vi "Read Simulation Sonar ID.vi"(5 "Ping DIO Channel":T1=enum."DIO 1", 9 "Echo DIO Channel":T1=enum."DIO 2") -> (8 "sonar ID":string, 10 "success?":bool)   [LabVIEW 2017]
uses:
  <vilib>/Rock Robotics/SystemInterfaces/DIO/FPGA_DIOChannel.ctl
panel:
  out "String":string
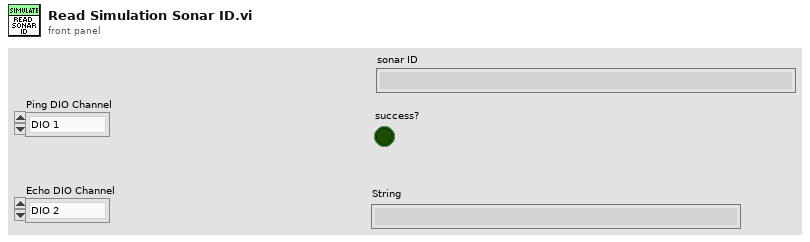
[diagram p1: front panel]
types:
  T1 = typedef "FPGA_DIOChannel.ctl" = enum8{"DIO 0", "DIO 1", "DIO 2", "DIO 3", "DIO 4", "DIO 5", "DIO 6", "DIO 7", "DIO 8", "DIO 9", "DIO MXP 0", "DIO MXP 1", "DIO MXP 2", "DIO MXP 3", "DIO MXP 4", "DIO MXP 5", "DIO MXP 6", "DIO MXP 7", "DIO MXP 8", "DIO MXP 9", "DIO MXP 10", "DIO MXP 11", "DIO MXP 12", "DIO MXP 13", "DIO MXP 14", "DIO MXP 15", "SPI Port CS1", "SPI Port CS2", "SPI Port CS3", "SPI Port MISO", "SPI Port MOSI", "Invalid"}
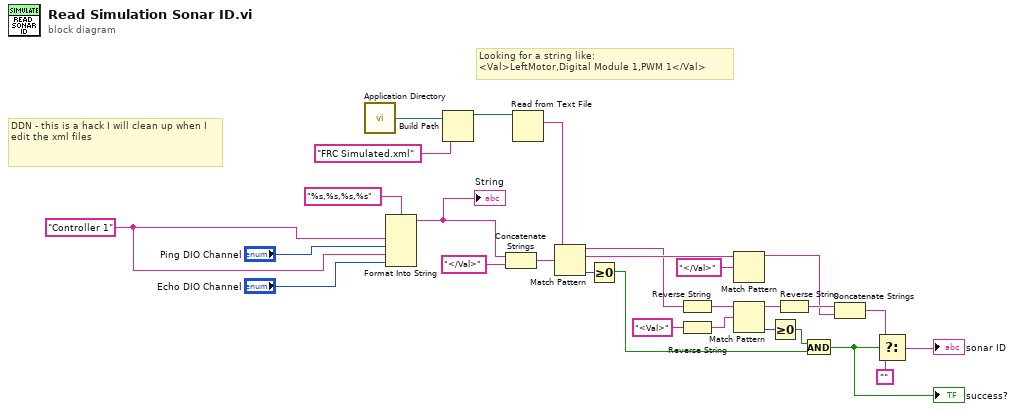
[diagram p0: block diagram]
diagram:
  w2 = "Controller 1" ("name or relative path")
  # "DDN - this is a hack I will clean up when I edit the xml files"
  # "Looking for a string like:\n<Val>LeftMotor,Digital Module 1,PWM 1</Val>"
  n1 = call <vilib>:"Application Directory.vi"() -> ("Application Directory"=w5:path)
  n2 = Format Into String(format string="%s,%s,%s,%s", w2, "Ping DIO Channel", w2, "Echo DIO Channel") -> (resulting string=w1:string)  [unwired: 2 in, 1 out]
  "String" <- w1
  n3 = Build Path(base path=w5, name or relative path="FRC Simulated.xml") -> (appended path=w23:path)
  n4 = Concatenate Strings(w1, "</Val>" ("name or relative path")) -> (w24:string)
  n5 = Read from Text File(file (use dialog)=w23) -> (text=w26:string)  [unwired: 3 in, 3 out]
  n6 = Match Pattern(string=w26, regular expression=w24) -> (before substring=w14:string, match substring=w18:string, offset past match=w12:i32)  [unwired: 1 in, 1 out]
  n7 = Greater Or Equal To 0?(x=w12) -> (x >= 0?=w10:bool)
  n8 = Reverse String(1:w14) -> (0:w22:string)
  n9 = Reverse String(1:"<Val>" ("name or relative path")) -> (0:w20:string)
  n10 = Match Pattern(string=w18, regular expression="</Val>" ("name or relative path")) -> (before substring=w15:string)  [unwired: 1 in, 3 out]
  n11 = Match Pattern(string=w22, regular expression=w20) -> (before substring=w19:string, offset past match=w13:i32)  [unwired: 1 in, 2 out]
  n12 = Greater Or Equal To 0?(x=w13) -> (x >= 0?=w11:bool)
  n13 = Reverse String(1:w19) -> (0:w16:string)
  n14 = And(x=w11, y=w10) -> (x .and. y?=w9:bool)
  "success?" <- w9
  n15 = Concatenate Strings(w16, w15) -> (w8:string)
  n16 = Select(t=w8, s=w9, f="") -> (s? t:f=→"sonar ID":string)
